vi "SVM_Model_Builder.vi"() -> ()   [LabVIEW 2014]
uses:
  <vilib>/Analysis/Matrix/Datatypes/RealMatrix.ctl
  <vilib>/Analysis/baseanly.llb/Real A x B.vi
  <vilib>/Utility/file.llb/Read From Spreadsheet File (DBL).vi
  <vilib>/Analysis/NI_AALBase.lvlib
  <vilib>/Analysis/Matrix/NI_Matrix.lvlib
panel:
  in  "MODEL_X4_Down movement":string="C:\\\\WORK\\\\MODEL_X4"
  in  "MODEL_X3_Up movement":string="C:\\\\WORK\\\\MODEL_X3"
  in  "MODEL_X2_Left movement":string="C:\\\\WORK\\\\MODEL_X2"
  in  "svm_parameter":T1={"svm_type"=0, "kernel_type"=2, "degree"=3, "gamma"=0.0, "coef0"=0.0, "cache_size"=40.0, "epsilon"=0.001, "C"=1000.0, "nr_weight"=0, "weight_label"=[1, -1], "Weight (C of class i)"=[1.0, 1.0], "nu"=0.5, "p"=0.1, "Shrinking"=1, "probability"=0} {"p" format="%.4f"; "nu" format="%.4f"; "Weight (C of class i)" format="%.2f"; "C" format="%.2f"; "epsilon" format="%.4f"; "cache_size" format="%.2f"; "coef0" format="%.2f"; "gamma" format="%.5f"; "kernel_type" items=["Linear", "Poly", "RBF", "Sigmoid"]; "svm_type" items=["C-SVC", "Nu-SVC", "One-class SVM", "epsilon-SVR", "nu-SVR"]}
  in  "MODEL_X1_Right movement":string="C:\\\\WORK\\\\MODEL_X1"
  out "X4":dbl[][](array[numeric]) format="%0.3f"
  out "X3":dbl[][](array[numeric]) format="%0.3f"
  out "X2":dbl[][](array[numeric]) format="%0.3f"
  out "X1":dbl[][](array[numeric]) format="%0.3f"
  out "WL4":T2
  out "WL3":T2
  out "WL2":T2
  out "WL1":T2
  in  "X4_Down movement":path
  in  "X3_Up movement":path
  in  "X2_Left movement":path
  in  "X1_Right movement":path
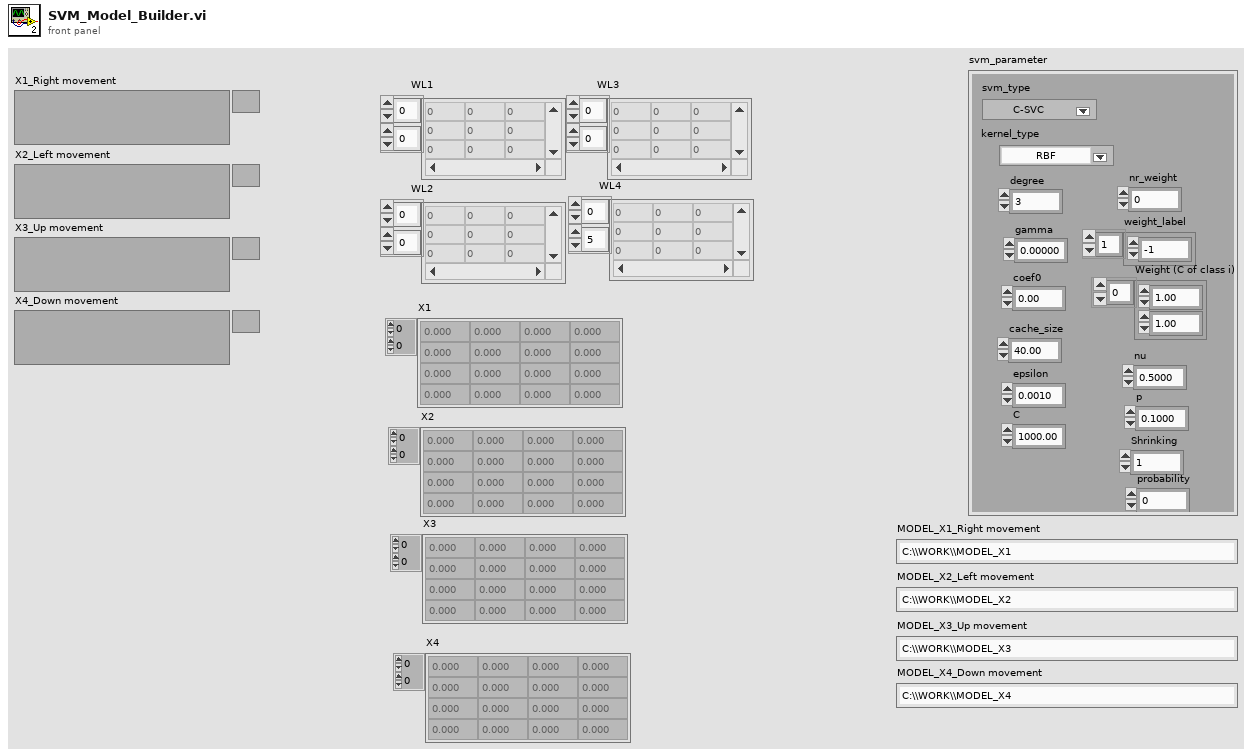
[diagram p1: front panel]
types:
  T1 = cluster{"svm_type":i16, "kernel_type":i16, "degree":i16, "gamma":dbl, "coef0":dbl, "cache_size":dbl, "epsilon":dbl, "C":dbl, "nr_weight":i16, "weight_label":i16[], "Weight (C of class i)":dbl[], "nu":dbl, "p":dbl, "Shrinking":i16, "probability":i16}
  T2 = typedef "NI_Matrix.lvlib/RealMatrix.ctl" = dbl[][]
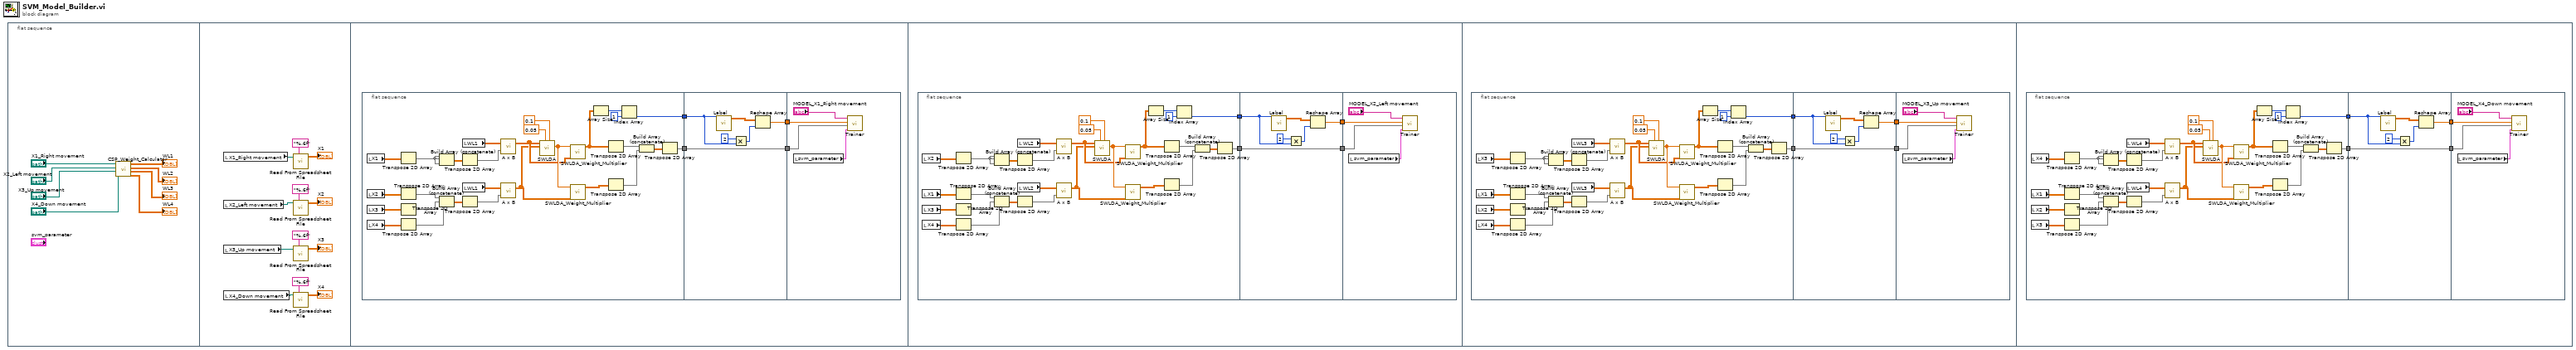
[diagram p0: block diagram]
diagram:
  n1 = flat-sequence {
    frame #0 {
      n2 = call "CSP_Weight_Calculator.vi"("X4_Down movement"="X4_Down movement", "X3_Up movement"="X3_Up movement", "X2_Left movement"="X2_Left movement", "X1_Right movement"="X1_Right movement") -> ("WL4"=→"WL4":T2, "WL3"=→"WL3":T2, "WL2"=→"WL2":T2, "WL1"=→"WL1":T2)  [unwired: 4 in]
    }
    frame #1 {
      n3 = local read "X1_Right movement"() -> (w20:path)
      n4 = local read "X2_Left movement"() -> (w15:path)
      n5 = local read "X3_Up movement"() -> (w14:path)
      n6 = local read "X4_Down movement"() -> (w13:path)
      n7 = call-poly <vilib>:"Read From Spreadsheet File.vi"("format (%.3f)"="%.6f", "file path (dialog if empty)"=w20) -> ("all rows"=→"X1":dbl[][])  [unwired: 5 in, 4 out]
      n8 = call-poly <vilib>:"Read From Spreadsheet File.vi"("format (%.3f)"="%.6f", "file path (dialog if empty)"=w15) -> ("all rows"=→"X2":dbl[][])  [unwired: 5 in, 4 out]
      n9 = call-poly <vilib>:"Read From Spreadsheet File.vi"("format (%.3f)"="%.6f", "file path (dialog if empty)"=w14) -> ("all rows"=→"X3":dbl[][])  [unwired: 5 in, 4 out]
      n10 = call-poly <vilib>:"Read From Spreadsheet File.vi"("format (%.3f)"="%.6f", "file path (dialog if empty)"=w13) -> ("all rows"=→"X4":dbl[][])  [unwired: 5 in, 4 out]
    }
    frame #2 {
      n11 = flat-sequence {
        tunnel: [w26] -> w24
        tunnel: [w25] -> w21
        tunnel: w24 -> [w55]
        tunnel: [w54] -> w23
        tunnel: [w53] -> w22
        tunnel: w21 -> [w53]
        tunnel: w23 -> [w62]
        tunnel: w22 -> [w61]
        frame #0 {
          n12 = local read "X1"() -> (w52:dbl[][])
          n13 = local read "X2"() -> (w51:dbl[][])
          n14 = local read "X3"() -> (w50:dbl[][])
          n15 = local read "X4"() -> (w49:dbl[][])
          n16 = Transpose 2D Array(2D array=w52) -> (transposed array=w48:dbl[][])
          n17 = Transpose 2D Array(2D array=w51) -> (transposed array=w47:dbl[][])
          n18 = Transpose 2D Array(2D array=w50) -> (transposed array=w46:dbl[][])
          n19 = Transpose 2D Array(2D array=w49) -> (transposed array=w45:dbl[][])
          n20 = Build Array (concatenate)(w48, w48, w48) -> (w44:dbl[][])
          n21 = Build Array (concatenate)(w47, w46, w45) -> (w43:dbl[][])
          n22 = local read "WL1"() -> (w42:T2)
          n23 = Transpose 2D Array(2D array=w44) -> (transposed array=w37:dbl[][])
          n24 = local read "WL1"() -> (w41:T2)
          n25 = Transpose 2D Array(2D array=w43) -> (transposed array=w40:dbl[][])
          n26 = call-poly <vilib>:"A x B.vi"("B"=w37, "A"=w42) -> ("A x B"=w35:T2)  [unwired: 1 out]
          n27 = call-poly <vilib>:"A x B.vi"("B"=w40, "A"=w41) -> ("A x B"=w34:T2)  [unwired: 1 out]
          n28 = call "SWLDA.vi"("premove"=0.1, "penter"=0.05, "ERP_Nontarget"=w34, "ERP_Target"=w35) -> ("WEIGHT"=w36:dbl[])  [unwired: 6 in, 1 out]
          n29 = call "SWLDA_Weight_Multiplier.vi"("Z_array"=w35, "Weight"=w36) -> ("CSP Processed\nSWSVM Array"=w27:dbl[][])  [unwired: 9 in]
          n30 = call "SWLDA_Weight_Multiplier.vi"("Z_array"=w34, "Weight"=w36) -> ("CSP Processed\nSWSVM Array"=w33:dbl[][])  [unwired: 9 in]
          n31 = Array Size(array=w27) -> (size(s)=w28:i32[])
          n32 = Transpose 2D Array(2D array=w27) -> (transposed array=w32:dbl[][])
          n33 = Transpose 2D Array(2D array=w33) -> (transposed array=w31:dbl[][])
          n34 = Index Array(array=w28, index=1) -> (element=w26:i32)
          n35 = Build Array (concatenate)(w32, w31) -> (w30:dbl[][])
          n36 = Transpose 2D Array(2D array=w30) -> (transposed array=w25:dbl[][])
        }
        frame #1 {
          n37 = call "Label.vi"("Numeric"=w55) -> ("Array"=w56:dbl[][])  [unwired: 10 in]
          n38 = Multiply(x=2, y=w55) -> (x*y=w58:i32)
          n39 = Reshape Array(w56, w58) -> (w54:dbl[])
        }
        frame #2 {
          n40 = local read "svm_parameter"() -> (w59:T1)
          n41 = call "Trainer.vi"("svm_parameter"=w59, "attributes"=w61, "Lables"=w62, "ModelFileName"="MODEL_X1_Right movement") -> ()
        }
      }
    }
    frame #3 {
      n42 = flat-sequence {
        tunnel: [w68] -> w66
        tunnel: [w67] -> w65
        tunnel: w66 -> [w97]
        tunnel: [w96] -> w64
        tunnel: [w95] -> w63
        tunnel: w65 -> [w95]
        tunnel: w64 -> [w104]
        tunnel: w63 -> [w103]
        frame #0 {
          n43 = local read "X2"() -> (w94:dbl[][])
          n44 = local read "X1"() -> (w93:dbl[][])
          n45 = local read "X3"() -> (w92:dbl[][])
          n46 = local read "X4"() -> (w91:dbl[][])
          n47 = Transpose 2D Array(2D array=w94) -> (transposed array=w90:dbl[][])
          n48 = Transpose 2D Array(2D array=w93) -> (transposed array=w89:dbl[][])
          n49 = Transpose 2D Array(2D array=w92) -> (transposed array=w88:dbl[][])
          n50 = Transpose 2D Array(2D array=w91) -> (transposed array=w87:dbl[][])
          n51 = Build Array (concatenate)(w90, w90, w90) -> (w86:dbl[][])
          n52 = Build Array (concatenate)(w89, w88, w87) -> (w85:dbl[][])
          n53 = local read "WL2"() -> (w84:T2)
          n54 = Transpose 2D Array(2D array=w86) -> (transposed array=w79:dbl[][])
          n55 = local read "WL2"() -> (w83:T2)
          n56 = Transpose 2D Array(2D array=w85) -> (transposed array=w82:dbl[][])
          n57 = call-poly <vilib>:"A x B.vi"("B"=w79, "A"=w84) -> ("A x B"=w77:T2)  [unwired: 1 out]
          n58 = call-poly <vilib>:"A x B.vi"("B"=w82, "A"=w83) -> ("A x B"=w76:T2)  [unwired: 1 out]
          n59 = call "SWLDA.vi"("premove"=0.1, "penter"=0.05, "ERP_Nontarget"=w76, "ERP_Target"=w77) -> ("WEIGHT"=w78:dbl[])  [unwired: 6 in, 1 out]
          n60 = call "SWLDA_Weight_Multiplier.vi"("Z_array"=w77, "Weight"=w78) -> ("CSP Processed\nSWSVM Array"=w69:dbl[][])  [unwired: 9 in]
          n61 = call "SWLDA_Weight_Multiplier.vi"("Z_array"=w76, "Weight"=w78) -> ("CSP Processed\nSWSVM Array"=w75:dbl[][])  [unwired: 9 in]
          n62 = Array Size(array=w69) -> (size(s)=w70:i32[])
          n63 = Transpose 2D Array(2D array=w69) -> (transposed array=w74:dbl[][])
          n64 = Transpose 2D Array(2D array=w75) -> (transposed array=w73:dbl[][])
          n65 = Index Array(array=w70, index=1) -> (element=w68:i32)
          n66 = Build Array (concatenate)(w74, w73) -> (w72:dbl[][])
          n67 = Transpose 2D Array(2D array=w72) -> (transposed array=w67:dbl[][])
        }
        frame #1 {
          n68 = call "Label.vi"("Numeric"=w97) -> ("Array"=w98:dbl[][])  [unwired: 10 in]
          n69 = Multiply(x=2, y=w97) -> (x*y=w100:i32)
          n70 = Reshape Array(w98, w100) -> (w96:dbl[])
        }
        frame #2 {
          n71 = local read "svm_parameter"() -> (w101:T1)
          n72 = call "Trainer.vi"("svm_parameter"=w101, "attributes"=w103, "Lables"=w104, "ModelFileName"="MODEL_X2_Left movement") -> ()
        }
      }
    }
    frame #4 {
      n73 = flat-sequence {
        tunnel: [w110] -> w108
        tunnel: [w109] -> w107
        tunnel: w108 -> [w139]
        tunnel: [w138] -> w106
        tunnel: [w137] -> w105
        tunnel: w107 -> [w137]
        tunnel: w106 -> [w146]
        tunnel: w105 -> [w145]
        frame #0 {
          n74 = local read "X3"() -> (w136:dbl[][])
          n75 = local read "X1"() -> (w135:dbl[][])
          n76 = local read "X2"() -> (w134:dbl[][])
          n77 = local read "X4"() -> (w133:dbl[][])
          n78 = Transpose 2D Array(2D array=w136) -> (transposed array=w132:dbl[][])
          n79 = Transpose 2D Array(2D array=w135) -> (transposed array=w131:dbl[][])
          n80 = Transpose 2D Array(2D array=w134) -> (transposed array=w130:dbl[][])
          n81 = Transpose 2D Array(2D array=w133) -> (transposed array=w129:dbl[][])
          n82 = Build Array (concatenate)(w132, w132, w132) -> (w128:dbl[][])
          n83 = Build Array (concatenate)(w131, w130, w129) -> (w127:dbl[][])
          n84 = local read "WL3"() -> (w126:T2)
          n85 = Transpose 2D Array(2D array=w128) -> (transposed array=w121:dbl[][])
          n86 = local read "WL3"() -> (w125:T2)
          n87 = Transpose 2D Array(2D array=w127) -> (transposed array=w124:dbl[][])
          n88 = call-poly <vilib>:"A x B.vi"("B"=w121, "A"=w126) -> ("A x B"=w119:T2)  [unwired: 1 out]
          n89 = call-poly <vilib>:"A x B.vi"("B"=w124, "A"=w125) -> ("A x B"=w118:T2)  [unwired: 1 out]
          n90 = call "SWLDA.vi"("premove"=0.1, "penter"=0.05, "ERP_Nontarget"=w118, "ERP_Target"=w119) -> ("WEIGHT"=w120:dbl[])  [unwired: 6 in, 1 out]
          n91 = call "SWLDA_Weight_Multiplier.vi"("Z_array"=w119, "Weight"=w120) -> ("CSP Processed\nSWSVM Array"=w111:dbl[][])  [unwired: 9 in]
          n92 = call "SWLDA_Weight_Multiplier.vi"("Z_array"=w118, "Weight"=w120) -> ("CSP Processed\nSWSVM Array"=w117:dbl[][])  [unwired: 9 in]
          n93 = Array Size(array=w111) -> (size(s)=w112:i32[])
          n94 = Transpose 2D Array(2D array=w111) -> (transposed array=w116:dbl[][])
          n95 = Transpose 2D Array(2D array=w117) -> (transposed array=w115:dbl[][])
          n96 = Index Array(array=w112, index=1) -> (element=w110:i32)
          n97 = Build Array (concatenate)(w116, w115) -> (w114:dbl[][])
          n98 = Transpose 2D Array(2D array=w114) -> (transposed array=w109:dbl[][])
        }
        frame #1 {
          n99 = call "Label.vi"("Numeric"=w139) -> ("Array"=w140:dbl[][])  [unwired: 10 in]
          n100 = Multiply(x=2, y=w139) -> (x*y=w142:i32)
          n101 = Reshape Array(w140, w142) -> (w138:dbl[])
        }
        frame #2 {
          n102 = local read "svm_parameter"() -> (w143:T1)
          n103 = call "Trainer.vi"("svm_parameter"=w143, "attributes"=w145, "Lables"=w146, "ModelFileName"="MODEL_X3_Up movement") -> ()
        }
      }
    }
    frame #5 {
      n104 = flat-sequence {
        tunnel: [w152] -> w150
        tunnel: [w151] -> w149
        tunnel: w150 -> [w181]
        tunnel: [w180] -> w148
        tunnel: [w179] -> w147
        tunnel: w149 -> [w179]
        tunnel: w148 -> [w188]
        tunnel: w147 -> [w187]
        frame #0 {
          n105 = local read "X4"() -> (w178:dbl[][])
          n106 = local read "X1"() -> (w177:dbl[][])
          n107 = local read "X2"() -> (w176:dbl[][])
          n108 = local read "X3"() -> (w175:dbl[][])
          n109 = Transpose 2D Array(2D array=w178) -> (transposed array=w174:dbl[][])
          n110 = Transpose 2D Array(2D array=w177) -> (transposed array=w173:dbl[][])
          n111 = Transpose 2D Array(2D array=w176) -> (transposed array=w172:dbl[][])
          n112 = Transpose 2D Array(2D array=w175) -> (transposed array=w171:dbl[][])
          n113 = Build Array (concatenate)(w174, w174, w174) -> (w170:dbl[][])
          n114 = Build Array (concatenate)(w173, w172, w171) -> (w169:dbl[][])
          n115 = local read "WL4"() -> (w168:T2)
          n116 = Transpose 2D Array(2D array=w170) -> (transposed array=w163:dbl[][])
          n117 = local read "WL4"() -> (w167:T2)
          n118 = Transpose 2D Array(2D array=w169) -> (transposed array=w166:dbl[][])
          n119 = call-poly <vilib>:"A x B.vi"("B"=w163, "A"=w168) -> ("A x B"=w161:T2)  [unwired: 1 out]
          n120 = call-poly <vilib>:"A x B.vi"("B"=w166, "A"=w167) -> ("A x B"=w160:T2)  [unwired: 1 out]
          n121 = call "SWLDA.vi"("premove"=0.1, "penter"=0.05, "ERP_Nontarget"=w160, "ERP_Target"=w161) -> ("WEIGHT"=w162:dbl[])  [unwired: 6 in, 1 out]
          n122 = call "SWLDA_Weight_Multiplier.vi"("Z_array"=w161, "Weight"=w162) -> ("CSP Processed\nSWSVM Array"=w153:dbl[][])  [unwired: 9 in]
          n123 = call "SWLDA_Weight_Multiplier.vi"("Z_array"=w160, "Weight"=w162) -> ("CSP Processed\nSWSVM Array"=w159:dbl[][])  [unwired: 9 in]
          n124 = Array Size(array=w153) -> (size(s)=w154:i32[])
          n125 = Transpose 2D Array(2D array=w153) -> (transposed array=w158:dbl[][])
          n126 = Transpose 2D Array(2D array=w159) -> (transposed array=w157:dbl[][])
          n127 = Index Array(array=w154, index=1) -> (element=w152:i32)
          n128 = Build Array (concatenate)(w158, w157) -> (w156:dbl[][])
          n129 = Transpose 2D Array(2D array=w156) -> (transposed array=w151:dbl[][])
        }
        frame #1 {
          n130 = call "Label.vi"("Numeric"=w181) -> ("Array"=w182:dbl[][])  [unwired: 10 in]
          n131 = Multiply(x=2, y=w181) -> (x*y=w184:i32)
          n132 = Reshape Array(w182, w184) -> (w180:dbl[])
        }
        frame #2 {
          n133 = local read "svm_parameter"() -> (w185:T1)
          n134 = call "Trainer.vi"("svm_parameter"=w185, "attributes"=w187, "Lables"=w188, "ModelFileName"="MODEL_X4_Down movement") -> ()
        }
      }
    }
  }
